vi "Toggle Auto Sort.vi"(8 "error in (no error)":errorcluster, 10 "Auto Sort":bool, 11 "List Data Type in":refnum<class "List Data Type.lvclass">) -> (0 "error out":errorcluster, 3 "List Data Type out":refnum<class "List Data Type.lvclass">)   [LabVIEW 2018, in "List Data Type.lvclass"]
uses:
  List Data Type.lvclass
  List Data Type.lvclass/List Data Type.ctl
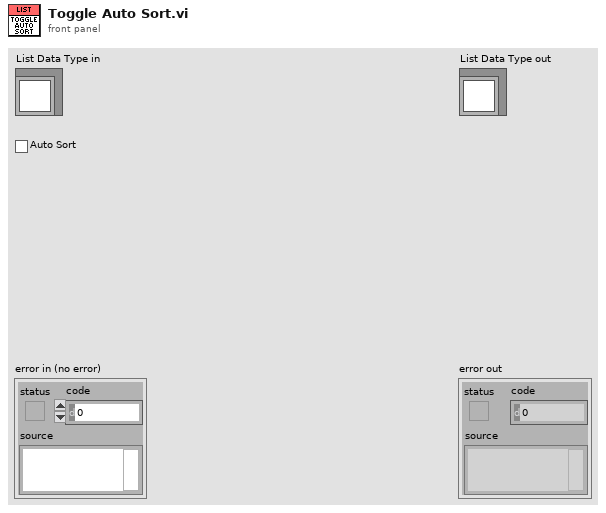
[diagram p1: front panel]
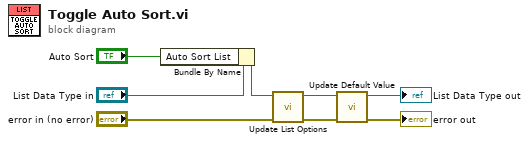
[diagram p0: block diagram]
diagram:
  n1 = Bundle By Name(cluster="List Data Type in", "Auto Sort List"="Auto Sort") -> (w6:refnum<class "List Data Type.lvclass">)
  n2 = call "Update List Options.vi"("error in (no error)"="error in (no error)", "List Data Type in"=w6) -> ("error out"=w3:errorcluster, "List Data Type out"=w5:refnum<class "List Data Type.lvclass">)  [unwired: 8 in]
  n3 = call "Update Default Value.vi"("error in (no error)"=w3, "List Data Type in"=w5) -> ("error out"=→"error out":errorcluster, "List Data Type out"=→"List Data Type out":refnum<class "List Data Type.lvclass">)  [unwired: 8 in]
